vi "Read pos_curr.vi"(8 "error in (no error)":errorcluster, 11 "smc100 in":refnum<class "smc100.lvclass">) -> (0 "error out":errorcluster, 2 "readback position":dbl[](array[numeric]), 3 "smc100 out":refnum<class "smc100.lvclass">)   [LabVIEW 2019, in "smc100.lvlib" / "smc100.lvclass"]
uses:
  smc100.lvclass
  smc100.lvclass/smc100.ctl
  Read VISA Handle.vi
  smc100.lvlib
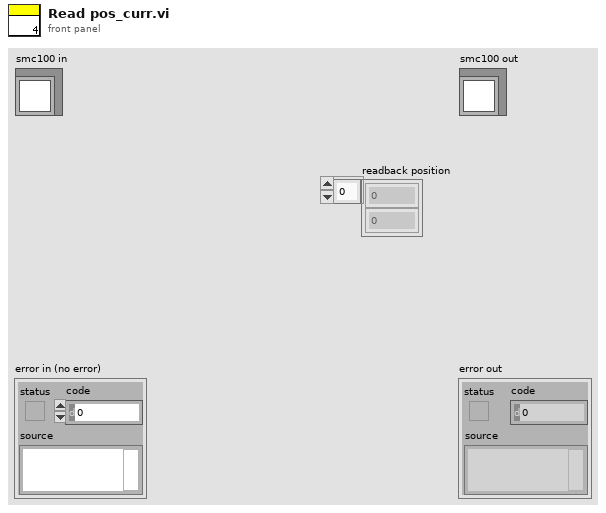
[diagram p1: front panel]
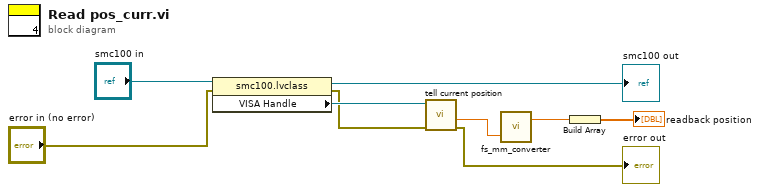
[diagram p0: block diagram]
diagram:
  n1 = property class="smc100.lvclass"(reference="smc100 in", error in="error in (no error)") -> (reference out=→"smc100 out":refnum<class "smc100.lvclass">, error out=w6:errorcluster, "VISA Handle"=w7:refnum<visa-resource-name>)
  n2 = call <userlib>:"tell current position.vi"("error in"=w6, "VISA Handle in"=w7) -> ("error out"=→"error out":errorcluster, "Current position (units)"=w2:dbl)  [unwired: 3 in, 3 out]
  n3 = call "fs_mm_converter.vi"("mm in"=w2) -> ("fs out"=w1:dbl)  [unwired: 1 in, 1 out]
  n4 = Build Array(w1) -> (→"readback position":dbl[])
